vi "Periodic Tasks.vi"(8 "error in":errorcluster) -> ()   [LabVIEW 2016]
doc: "This VI runs in parallel to other tasks. It can contain as many user-defined periodic loops as you need. These can carry out PID or other sorts of timed response."
uses:
  <vilib>/Rock Robotics/WPI/Solenoid/WPI_SolenoidValue.ctl
  <vilib>/Rock Robotics/WPI/Utilities/WPI_GetSetVariantRefNum.vi
  Robot Global Data.vi
  <vilib>/addons/control/pid/pid.llb/PID (DBL).vi
  <vilib>/Rock Robotics/WPI/RobotDrive/WPI_RobotDriveMecanumDrive_Cartesian.vi
  <vilib>/Rock Robotics/WPI/Solenoid/WPI_SolenoidSetEnum.vi
  <vilib>/Rock Robotics/Network Tables/NT Read Number.vi
  <vilib>/Rock Robotics/Network Tables/NT Write Boolean.vi
  <vilib>/Rock Robotics/Network Tables/NT Write Number.vi
  <vilib>/Rock Robotics/Network Tables/NT Read Numeric Array.vi
  navX Library v2/navX Library v2.lvlib
  <vilib>/addons/control/pid/NI_PID_pid.lvlib
panel:
  out "timeSaved convey":i32
  out "timeSaved gears":i32
  out "encXsaved":dbl
  out "encYsaved":dbl
  out "voltage dash":dbl=12.55
  out "shooting far":bool
  out "shooting close":bool
  out "kill compress shoot":bool
  out "Pitch":dbl=0.2
  out "target angle":dbl=-4.022499999999997
  in  "cam FOV":dbl=34.0 format="%#_13g"
  out "YavSaved":dbl=-21.13
  in  "min thresh":dbl=5e-05 format="%#_13g"
  in  "add if slow":dbl=0.005 format="%#_13g"
  in  "add if fast":dbl format="%#_13g"
  out "turnSpeedSlow working":dbl=0.18
  out "aimState":i32
  out "leftOrRight":dbl=1.0
  out "aimBot":dbl
  in  "SEQ Retainer Open":bool
  in  "Gear Shover":bool
  in  "Ramp-Up":dbl format="%#_13g"
  out "Shooter Speed":dbl=-0.0
  out "trim close":dbl=0.9968503937007874
  out "trim far":dbl=1.0
  out "timeSaved 2":i32=29435
  out "timeSaved":i32=46200
  in  "Slews":cluster{"slewX":dbl, "slewY":dbl, "slewZ":dbl}={"slewX"=0.2, "slewY"=0.2, "slewZ"=0.15}
  # "ANYTHING AND EVERYTHING AUTOAIM"
  # "DRIVE STUFF"
  # "BALL STUFF"
  # "GEAR STUFF"
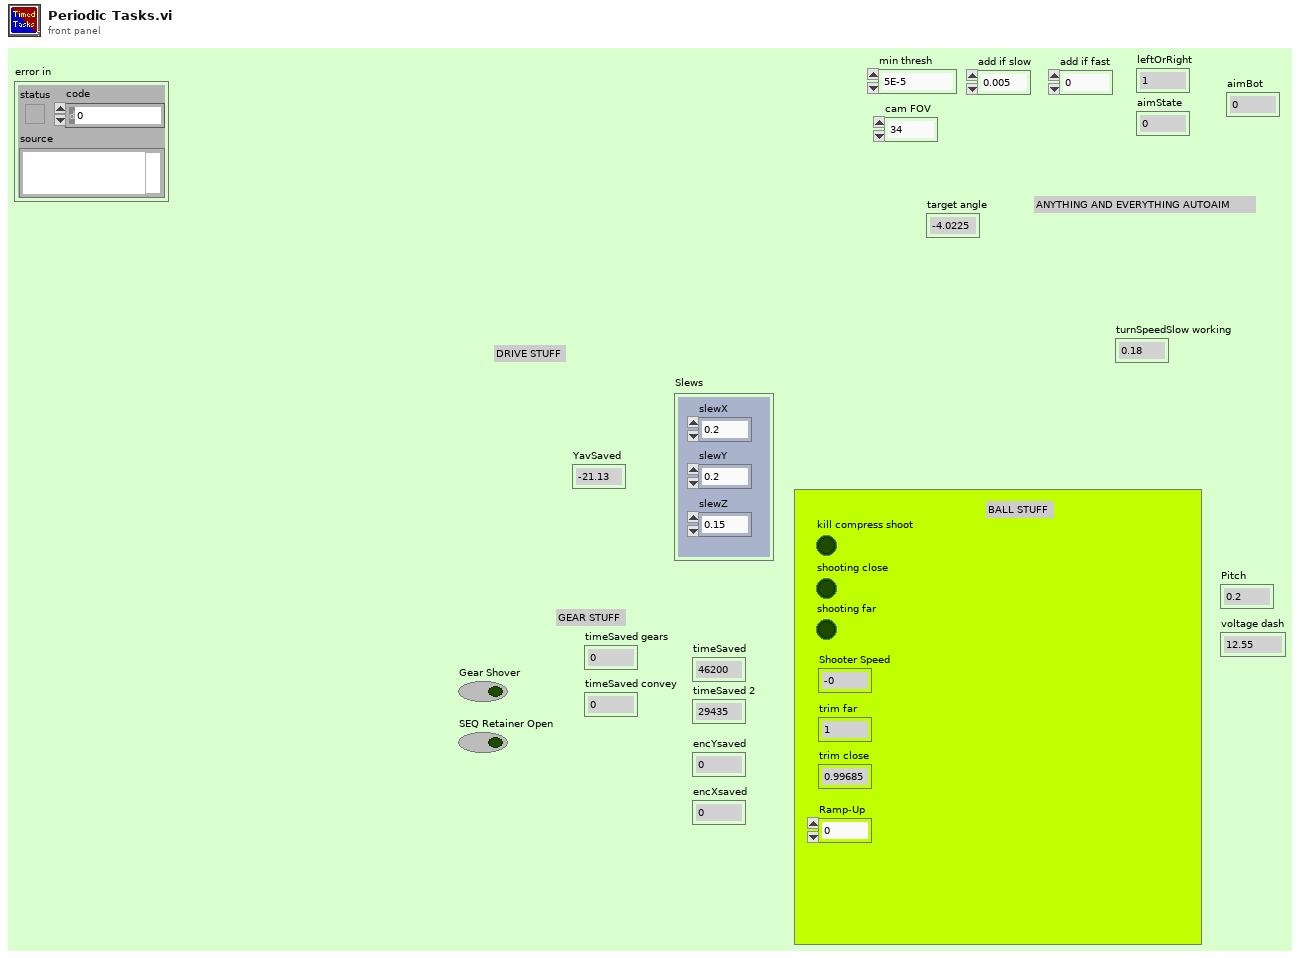
[diagram p1: front panel]
types:
  T1 = typedef "WPI_MotorControlDeviceRef.ctl" = cluster{"DeviceStatus":errorcluster, "Type":T2, "PWM":cluster{"PWM Channel":T3, "DeadBand":T4}, "CAN":cluster{"Device Number":u8, "SetOutput VI Ref":variant, "GetOutput VI Ref":variant, "Enable VI Ref":variant, "Disable VI Ref":variant, "Data":variant}, "Invert":bool}
  T2 = typedef "WPI_MotorControlType.ctl" = enum16{"PWM", "CAN"}
  T3 = typedef "FPGA_DIOPWMChannel.ctl" = enum8{"PWM 0", "PWM 1", "PWM 2", "PWM 3", "PWM 4", "PWM 5", "PWM 6", "PWM 7", "PWM 8", "PWM 9", "PWM MXP 0", "PWM MXP 1", "PWM MXP 2", "PWM MXP 3", "PWM MXP 4", "PWM MXP 5", "PWM MXP 6", "PWM MXP 7", "PWM MXP 8", "PWM MXP 9", "Invalid"}
  T4 = typedef "WPI_PWMDeadband.ctl" = cluster{"Name":string, "maxPositivePwm":i32, "minPositivePwm":i32, "centerPwm":i32, "maxNegativePwm":i32, "minNegativePwm":i32, "angularRange":u16}
  T5 = typedef "WPI_SolenoidDevRef.ctl" = cluster{"DevStatus":errorcluster, "Pneumatics Control Module":u8, "Forward Solenoid Channel":T6, "Reverse Solenoid Channel":T6}
  T6 = typedef "WPI_SolenoidChannel.ctl" = enum8{"Solenoid 0", "Solenoid 1", "Solenoid 2", "Solenoid 3", "Solenoid 4", "Solenoid 5", "Solenoid 6", "Solenoid 7", "Invalid"}
  T7 = typedef "WPI_CompressorDevRef.ctl" = cluster{"DevStatus":errorcluster, "Pneumatics Control Module":u8}
  T8 = typedef "WPI_ServoDeviceRef.ctl" = cluster{"DeviceStatus":errorcluster, "PWM Channel":T3, "DeadBand":T4}
  T9 = typedef "WPI_RobotDriveDevRef.ctl" = cluster{"DevStatus":errorcluster, "Motors[]":T1[], "Square Inputs":bool, "Max Output":dbl}
  T10 = typedef "navX Library v2.lvlib/Z900_navX_DeviceTypeDef.ctl" = cluster{"Interface":cluster{"Protocol":T11, "Update Rate (4Hz-100Hz)":u8, "navX Open TypeDef":variant}, "Notify Packet":refnum<notifier>, "Loop VI Refnum":refnum<vi>, "Ready to Close Occurrence Refnum":refnum<k4>}
  T11 = typedef "navX Library v2.lvlib/Z900_navX_ProtocolTypeDef.ctl" = enum16{"SERIAL", "I2C", "SPI"}
  T12 = typedef "WPI_SolenoidValue.ctl" = enum16{"Off", "On", "Forward", "Reverse"}
  T13 = typedef "WPI_EncoderDevRef.ctl" = cluster{"DevStatus":errorcluster, "EncoderIndex":T14, "CounterIndex":T15, "DistancePerCount":dbl, "Decoding Type":T16}
  T14 = typedef "FPGA_EncoderIdx.ctl" = enum8{"Enc 0", "Enc 1", "Enc 2", "Enc 3", "Enc 4", "Enc 5", "Enc 6", "Enc 7", "Invalid"}
  T15 = typedef "FPGA_CounterCtrSystemIndex.ctl" = enum8{"Ctr 0", "Ctr 1", "Ctr 2", "Ctr 3", "Ctr 4", "Ctr 5", "Ctr 6", "Ctr 7", "Invalid"}
  T16 = typedef "WPI_EncoderType.ctl" = enum16{"1x", "2x", "4x"}
  T17 = typedef "WPI_DriverStationRobotMode2.ctl" = enum16{"Autonomous Disabled", "Autonomous Enabled", "Teleop Disabled", "Teleop Enabled", "Disconnected", "Finish", "Test Disabled", "Test Enabled", "Emergency Stopped"}
  T18 = cluster{"proportional gain (Kc)":dbl, "integral time (Ti, min)":dbl, "derivative time (Td, min)":dbl}
  T19 = cluster{"Yaw":dbl, "Roll":dbl, "Pitch":dbl, "Heading":dbl, "Fused Heading":dbl}
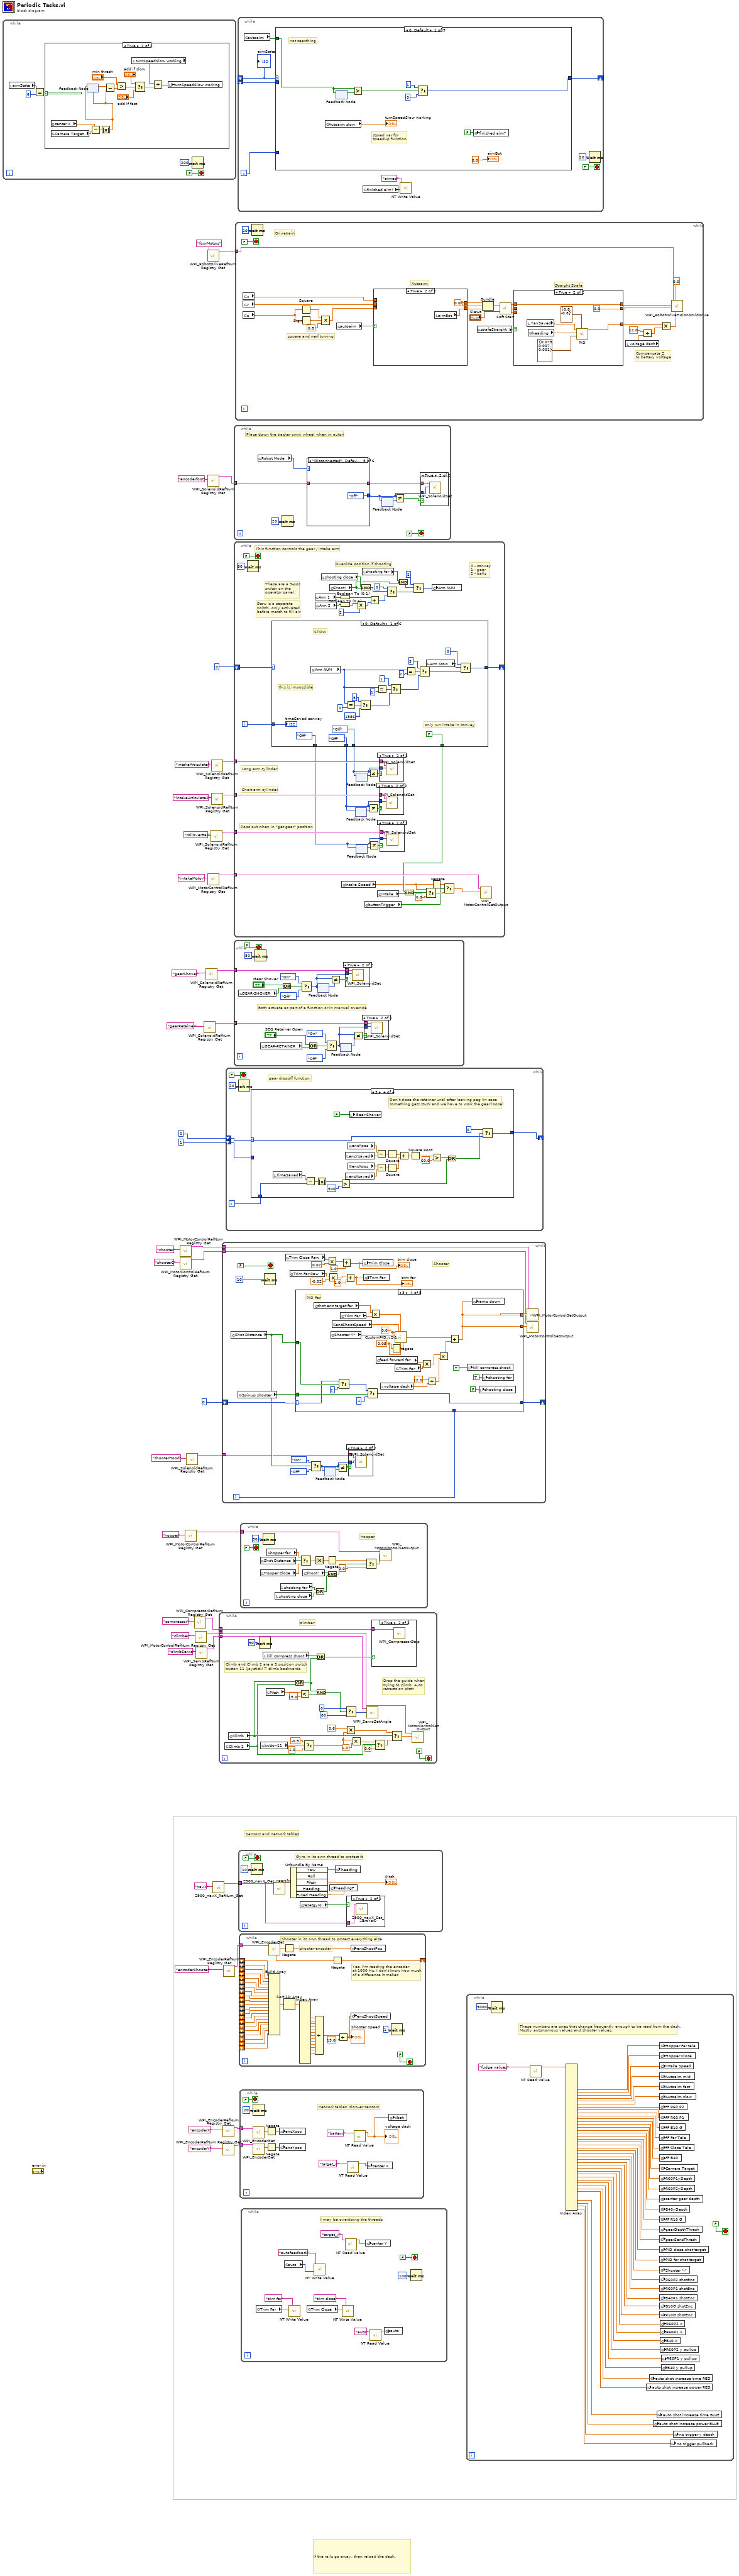
[diagram p0: block diagram]
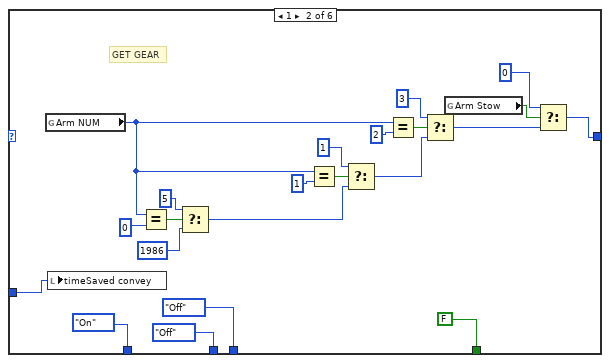
[diagram p5: hidden frame]
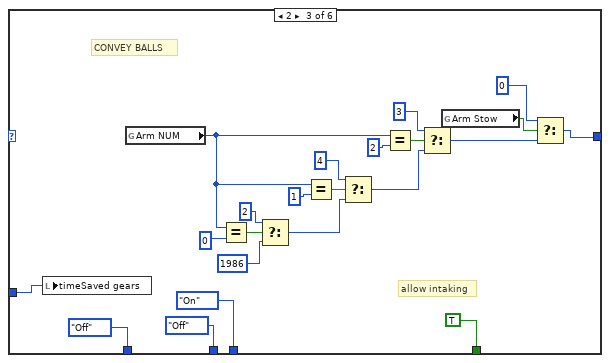
[diagram p6: hidden frame]
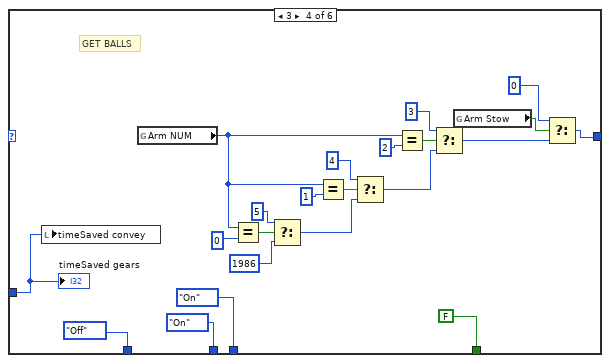
[diagram p7: hidden frame]
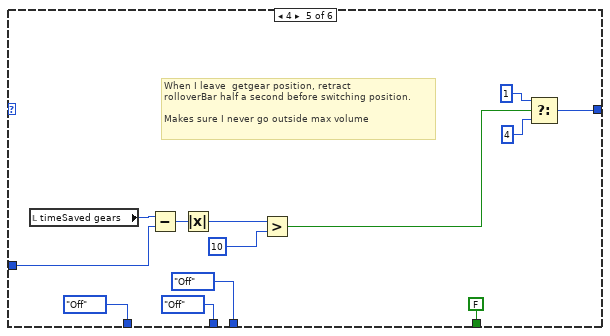
[diagram p8: hidden frame]
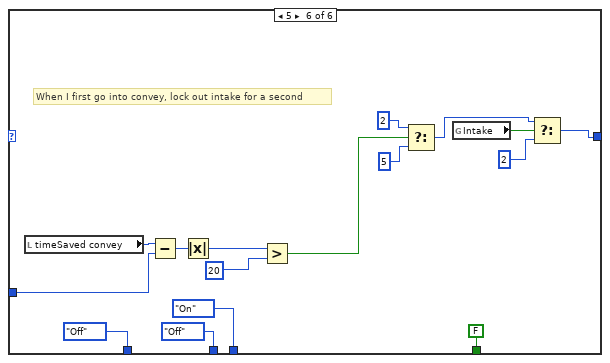
[diagram p9: hidden frame]
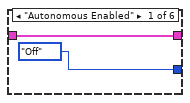
[diagram p11: hidden frame]
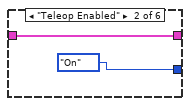
[diagram p12: hidden frame]
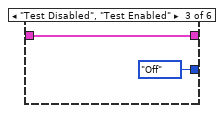
[diagram p13: hidden frame]
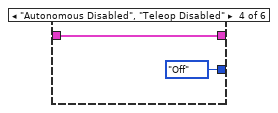
[diagram p14: hidden frame]
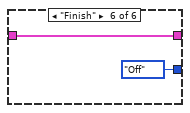
[diagram p15: hidden frame]
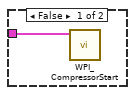
[diagram p17: hidden frame]
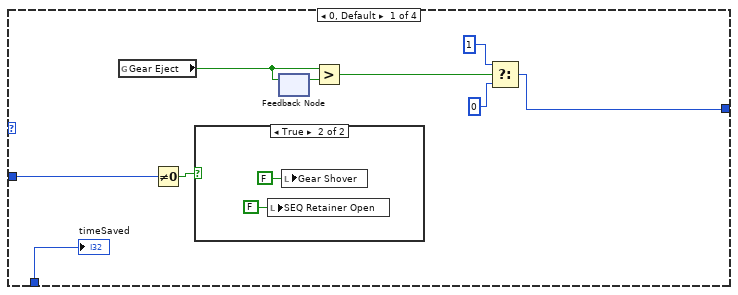
[diagram p18: hidden frame]
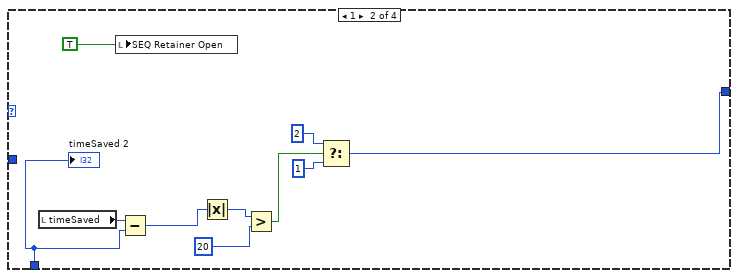
[diagram p20: hidden frame]
diagram:
  # "Sensors and network tables"
  # "If the rails go away, then reload the dash."
  n1 = while {
    stop <- FALSE stop-if-true
    n2 = local read "aimState"() -> (w45:i32)
    n3 = Equal?(x=w45, y=6) -> (x = y?=w43:bool)
    n4 = case shown="True" w43 {
      frame False {
      }
      frame True {
        n5 = global read "Robot Global Data.vi" "center X"() -> (w60:dbl)
        n6 = global read "Robot Global Data.vi" "Camera Target"() -> (w48:dbl)
        n7 = Subtract(x=w60, y=w48) -> (x-y=w50:dbl)
        n8 = Absolute Value(x=w50) -> (abs(x)=w49:dbl)
        n9 = feedback #1(w49) -> (w58:dbl)
        n10 = feedback-in #1(w49) -> ()
        n11 = Subtract(x=w58, y=w49) -> (x-y=w57:dbl)
        n12 = Greater?(x="min thresh", y=w57) -> (0:w55:bool)
        n13 = local read "turnSpeedSlow working"() -> (w52:dbl)
        n14 = Select(t="add if slow", s=w55, f="add if fast") -> (s? t:f=w53:dbl)
        n15 = Add(x=w52, y=w53) -> (x+y=w51:dbl)
        n16 = local write "turnSpeedSlow working"(w51) -> ()
      }
    }
    n17 = Wait (ms)(milliseconds to wait=u32 200) -> ()  [unwired: 1 out]
  }
  n18 = call <vilib>:"WPI_MotorControlRefNum Registry Get.vi"("refnum name"="shooter") -> ("MotorControlDevRef"=w31:T1)  [unwired: 9 in, 1 out]
  n19 = call <vilib>:"WPI_MotorControlRefNum Registry Get.vi"("refnum name"="shooter2") -> ("MotorControlDevRef"=w30:T1)  [unwired: 9 in, 1 out]
  n20 = call <vilib>:"WPI_MotorControlRefNum Registry Get.vi"("refnum name"="hopper") -> ("MotorControlDevRef"=w28:T1)  [unwired: 9 in, 1 out]
  n21 = call <vilib>:"WPI_SolenoidRefNum Registry Get.vi"("refnum name"="shooterHood") -> ("SolenoidDevRef"=w32:T5)  [unwired: 9 in, 1 out]
  n22 = call <vilib>:"WPI_CompressorRefNum Registry Get.vi"("refnum name"="compressor") -> ("CompressorDevRef"=w1:T7)  [unwired: 9 in, 1 out]
  n23 = call <vilib>:"WPI_MotorControlRefNum Registry Get.vi"("refnum name"="climber") -> ("MotorControlDevRef"=w24:T1)  [unwired: 9 in, 1 out]
  n24 = call <vilib>:"WPI_ServoRefNum Registry Get.vi"("refnum name"="climbServo") -> ("ServoDeviceRef"=w14:T8)  [unwired: 9 in, 1 out]
  n25 = call <vilib>:"WPI_SolenoidRefNum Registry Get.vi"("refnum name"="gearRetainer") -> ("SolenoidDevRef"=w37:T5)  [unwired: 9 in, 1 out]
  n26 = call <vilib>:"WPI_SolenoidRefNum Registry Get.vi"("refnum name"="gearShover") -> ("SolenoidDevRef"=w38:T5)  [unwired: 9 in, 1 out]
  n27 = call <vilib>:"WPI_RobotDriveRefNum Registry Get.vi"("refnum name"="fourMotors") -> ("RobotDriveDevRef"=w41:T9)  [unwired: 1 in, 9 out]
  n28 = call <vilib>:"WPI_SolenoidRefNum Registry Get.vi"("refnum name"="encoderfoot") -> ("SolenoidDevRef"=w11:T5)  [unwired: 9 in, 1 out]
  n29 = call <vilib>:"WPI_MotorControlRefNum Registry Get.vi"("refnum name"="intakeMotor") -> ("MotorControlDevRef"=w4:T1)  [unwired: 9 in, 1 out]
  n30 = call <vilib>:"WPI_SolenoidRefNum Registry Get.vi"("refnum name"="rolloverBar") -> ("SolenoidDevRef"=w2:T5)  [unwired: 9 in, 1 out]
  n31 = call <vilib>:"WPI_SolenoidRefNum Registry Get.vi"("refnum name"="intakeArticulate") -> ("SolenoidDevRef"=w8:T5)  [unwired: 9 in, 1 out]
  n32 = call <vilib>:"WPI_SolenoidRefNum Registry Get.vi"("refnum name"="intakeArticulate2") -> ("SolenoidDevRef"=w6:T5)  [unwired: 9 in, 1 out]
  n33 = call "Z900_navX_RefNum_Get.vi"("refnum name"="navX") -> ("navX Device"=w22:T10)  [unwired: 9 in, 1 out]
  n34 = while {
    tunnel: w24 -> [w67]
    tunnel: w14 -> [w83]
    tunnel: w1 -> [w75]
    stop <- FALSE stop-if-true
    # "Drop the guide when\ntrying to climb. Auto\nretracts on pitch"
    # "Climb and Climb 2 are a 3 position switch\nbutton 11 (joystick) = climb backwards"
    # "climber"
    n35 = global read "Robot Global Data.vi" "Climb 2"() -> (w64:bool)
    n36 = global read "Robot Global Data.vi" "Climb"() -> (w63:bool)
    n37 = Wait (ms)(milliseconds to wait=u32 50) -> ()  [unwired: 1 out]
    n38 = global read "Robot Global Data.vi" "button11"() -> (w69:bool)
    n39 = local read "kill compress shoot"() -> (w66:bool)
    n40 = local read "Pitch"() -> (w79:dbl)
    n41 = Or(x=w63, y=w64) -> (x .or. y?=w65:bool)
    n42 = Less?(x=w79, y=15.0) -> (x < y?=w80:bool)
    n43 = Select(t=-0.5, s=w69, f=1.0) -> (s? t:f=w61:dbl)
    n44 = Or(x=w66, y=w65) -> (x .or. y?=w76:bool)
    n45 = And(x=w65, y=w80) -> (x .and. y?=w77:bool)
    n46 = Select(t=0 ("servo down angle"), s=w77, f=80 ("servo up angle")) -> (s? t:f=w84:i32)
    n47 = Multiply(x=0.6 ("climb slow"), y=w61) -> (x*y=w68:dbl)
    n48 = Multiply(x=w61, y=1.0 ("t")) -> (x*y=w71:dbl)
    n49 = call <vilib>:"WPI_ServoSetAngle.vi"("Angle"=w84, "ServoDeviceRef"=w83) -> ()  [unwired: 8 in, 2 out]
    n50 = case shown="True" w76 {
      tunnel: w75 -> [w89 w90]
      frame False {
        n51 = call <vilib>:"WPI_CompressorStart.vi"("CompressorDevRef"=w89) -> ()  [unwired: 9 in, 2 out]
      }
      frame True {
        n52 = call <vilib>:"WPI_CompressorStop.vi"("CompressorDevRef"=w90) -> ()  [unwired: 9 in, 2 out]
      }
    }
    n53 = Select(t=w71, s=w64, f=0.0) -> (s? t:f=w85:dbl)
    n54 = Select(t=w68, s=w63, f=w85) -> (s? t:f=w74:dbl)
    n55 = call <vilib>:"WPI_MotorControlSetOutput.vi"("Output"=w74, "MotorControlDevRef"=w67) -> ()  [unwired: 7 in, 3 out]
  }
  n56 = while {
    shift-right: [w113] -> _
    shift-left: 0 ("y") -> [w115]
    tunnel: w32 -> [w96]
    tunnel: w31 -> [w95]
    tunnel: w30 -> [w94]
    i -> [w91]
    stop <- FALSE stop-if-true
    # "Shooter"
    n57 = global read "Robot Global Data.vi" "Shot Distance"() -> (w97:bool)
    n58 = global read "Robot Global Data.vi" "Spinup shooter"() -> (w114:bool)
    n59 = Wait (ms)(milliseconds to wait=u32 10) -> ()  [unwired: 1 out]
    n60 = global read "Robot Global Data.vi" "Trim Close Raw"() -> (w104:dbl)
    n61 = global read "Robot Global Data.vi" "Trim Far Raw"() -> (w106:dbl)
    n62 = case shown="3" w115 {
      selector: w115 -> [_ _ w167 w193 _]
      tunnel: w114 -> [w125 w143 w171 w192 _]
      tunnel: [w126 w139 w165 w191 w203] -> w113
      tunnel: [w122 w133 w156 w181 w200] -> w112
      tunnel: [w122 w133 w156 w181 w200] -> w111
      tunnel: w97 -> [_ w129 w168 w195 _]
      tunnel: w91 -> [_ _ _ _ _]
      frame 0, Default {
        w120 = FALSE ("shooting far")
        w122 = 0.0
        # "1"
        # "Reset Ramp to 0"
        # "Shooter-off"
        n63 = local write "Ramp-Up"(0.0 ("Power")) -> ()
        n64 = Select(t=1 ("f"), s=w125, f=0 ("y")) -> (s? t:f=w126:i32)
        "kill compress shoot" <- FALSE ("kill compress shoot")
        "shooting close" <- w120
        "shooting far" <- w120
      }
      frame 1 {
        # "Limit shooter spinup\n(should take ~1 sec"
        n65 = global read "Robot Global Data.vi" "FF Close Tele"() -> (w132:dbl)
        n66 = global read "Robot Global Data.vi" "feed forward far"() -> (w130:dbl)
        n67 = Add(x=0.01, y="Ramp-Up") -> (x+y=w133:dbl)
        n68 = local write "Ramp-Up"(w133) -> ()
        n69 = Select(t=w130, s=w129, f=w132) -> (s? t:f=w131:dbl)
        n70 = Select(t=1 ("f"), s=w143, f=4 ("y")) -> (s? t:f=w141:i32)
        n71 = Greater Or Equal?(x=w133, y=w131) -> (x >= y?=w140:bool)
        n72 = Select(t=3 ("y"), s=w129, f=2 ("y")) -> (s? t:f=w134:i32)
        n73 = Select(t=w134, s=w140, f=w141) -> (s? t:f=w139:i32)
        n74 = global write "Robot Global Data.vi" "ramp down"(w133) -> ()
        n75 = local write "kill compress shoot"(TRUE ("kill compress shoot")) -> ()
      }
      frame 2 {
        w147 = 0.0 ("Kp")
        w145 = 0.05 ("Max Ouput")
        # "PID Close"
        n76 = global read "Robot Global Data.vi" "PID close shot target"() -> (w152:dbl)
        n77 = global read "Robot Global Data.vi" "Shooter \"i\""() -> (w153:dbl)
        n78 = Select(t=3, s=w168, f=w167) -> (s? t:f=w166:i32)
        n79 = global read "Robot Global Data.vi" "Trim Close"() -> (w161:dbl)
        n80 = global read "Robot Global Data.vi" "encShootSpeed"() -> (w150:dbl)
        n81 = Select(t=w166, s=w171, f=4) -> (s? t:f=w165:i32)
        n82 = global read "Robot Global Data.vi" "FF Close Tele"() -> (w154:dbl)
        n83 = global read "Robot Global Data.vi" "Trim Close"() -> (w158:dbl)
        n84 = Multiply(x=w152, y=w161) -> (x*y=w160:dbl)
        n85 = local read "voltage dash"() -> (w155:dbl)
        n86 = Negate(x=w145) -> (-x=w146:dbl)
        n87 = call "CustomPID_v2.1.vi"("Kp"=w147, "Process Variable"=w150, "Goal"=w160, "Ki"=w153, "Kd"=w147, "Max Ouput"=w145, "Min Output"=w146) -> ("Command"=w159:dbl)  [unwired: 6 in, 2 out]
        n88 = Multiply(x=w154, y=w158) -> (x*y=w157:dbl)
        n89 = Divide(x=12.0, y=w155) -> (x/y=w163:dbl)
        n90 = Multiply(x=w157, y=w163) -> (x*y=w162:dbl)
        n91 = Add(x=w159, y=w162) -> (x+y=w156:dbl)
        n92 = local write "kill compress shoot"(TRUE ("kill compress shoot")) -> ()
        n93 = global write "Robot Global Data.vi" "ramp down"(w156) -> ()
        n94 = local write "shooting far"(FALSE ("shooting far")) -> ()
        n95 = local write "shooting close"(TRUE ("shooting close")) -> ()
      }
      frame 3 {
        w174 = 0.0 ("Kp")
        w172 = 0.05 ("Max Ouput")
        # "PID Far"
        n96 = global read "Robot Global Data.vi" "shot enc target far"() -> (w177:dbl)
        n97 = global read "Robot Global Data.vi" "Shooter \"i\""() -> (w179:dbl)
        n98 = global read "Robot Global Data.vi" "encShootSpeed"() -> (w185:dbl)
        n99 = Select(t=w193, s=w195, f=2 ("t")) -> (s? t:f=w196:i32)
        n100 = global read "Robot Global Data.vi" "Trim Far"() -> (w198:dbl)
        n101 = Select(t=w196, s=w192, f=4) -> (s? t:f=w191:i32)
        n102 = Multiply(x=w177, y=w198) -> (x*y=w186:dbl)
        n103 = global read "Robot Global Data.vi" "feed forward far"() -> (w182:dbl)
        n104 = local read "voltage dash"() -> (w180:dbl)
        n105 = Negate(x=w172) -> (-x=w173:dbl)
        n106 = call "CustomPID_v2.1.vi"("Kp"=w174, "Process Variable"=w185, "Goal"=w186, "Ki"=w179, "Kd"=w174, "Max Ouput"=w172, "Min Output"=w173) -> ("Command"=w187:dbl)  [unwired: 6 in, 2 out]
        n107 = global read "Robot Global Data.vi" "Trim Far"() -> (w184:dbl)
        n108 = Multiply(x=w182, y=w184) -> (x*y=w183:dbl)
        n109 = Divide(x=12.0, y=w180) -> (x/y=w189:dbl)
        n110 = Multiply(x=w183, y=w189) -> (x*y=w188:dbl)
        n111 = Add(x=w187, y=w188) -> (x+y=w181:dbl)
        n112 = local write "kill compress shoot"(TRUE ("kill compress shoot")) -> ()
        n113 = global write "Robot Global Data.vi" "ramp down"(w181) -> ()
        n114 = local write "shooting close"(FALSE ("shooting close")) -> ()
        n115 = local write "shooting far"(TRUE ("shooting far")) -> ()
      }
      frame 4 {
        # "With coast mode this is probably unecessary, but I left it in because I don't want to risk it\nI mean, we do cut the shooter abrubptly at the end of auto,="
        n116 = global read "Robot Global Data.vi" "ramp down"() -> (w201:dbl)
        n117 = Add(x=-0.002, y=w201) -> (x+y=w200:dbl)
        n118 = global write "Robot Global Data.vi" "ramp down"(w200) -> ()
        n119 = Less Or Equal To 0?(x=w200) -> (x <= 0?=w202:bool)
        n120 = Select(t=0 ("f"), s=w202, f=4 ("y")) -> (s? t:f=w203:i32)
        n121 = local write "kill compress shoot"(FALSE ("kill compress shoot")) -> ()
      }
    }
    n122 = Select(t=WPI_SolenoidValue."On" ("Value"), s=w97, f=WPI_SolenoidValue."Off" ("Value")) -> (s? t:f=w102:T12)
    n123 = feedback #2() -> (w100:T12)  [unwired: 1 in]
    n124 = feedback-in #2(w102) -> ()
    n125 = Multiply(x=w104, y=0.02 ("value")) -> (x*y=w107:dbl)
    n126 = Multiply(x=w106, y=-0.02 ("value")) -> (x*y=w110:dbl)
    n127 = Not Equal?(x=w102, y=w100) -> (x != y?=w101:bool)
    n128 = Add(x=w107, y=1.0) -> (x+y=w92:dbl)
    "trim close" <- w92
    n129 = Add(x=w110, y=1.0) -> (x+y=w93:dbl)
    "trim far" <- w93
    n130 = case shown="True" w101 {
      tunnel: w102 -> [_ w119]
      tunnel: w96 -> [_ w118]
      frame False {
      }
      frame True {
        n131 = call-poly <vilib>:"WPI_SolenoidSet.vi"("Value"=w119, "SolenoidDevRef"=w118) -> ()  [unwired: 8 in, 2 out]
      }
    }
    n132 = global write "Robot Global Data.vi" "Trim Close"(w92) -> ()
    n133 = global write "Robot Global Data.vi" "Trim Far"(w93) -> ()
    n134 = call <vilib>:"WPI_MotorControlSetOutput.vi"("Output"=w112, "MotorControlDevRef"=w95) -> ()  [unwired: 7 in, 3 out]
    n135 = call <vilib>:"WPI_MotorControlSetOutput.vi"("Output"=w111, "MotorControlDevRef"=w94) -> ()  [unwired: 7 in, 3 out]
  }
  n136 = call <vilib>:"WPI_EncoderRefNum Registry Get.vi"("refnum name"="encoderX") -> ("EncoderDevRef"=w18:T13)  [unwired: 9 in, 1 out]
  n137 = call <vilib>:"WPI_EncoderRefNum Registry Get.vi"("refnum name"="encoderY") -> ("EncoderDevRef"=w16:T13)  [unwired: 9 in, 1 out]
  n138 = call <vilib>:"WPI_EncoderRefNum Registry Get.vi"("refnum name"="encoderShooter") -> ("EncoderDevRef"=w20:T13)  [unwired: 9 in, 1 out]
  n139 = while {
    shift-right: [w209] -> _
    shift-left: 0 ("f") -> [w210]
    shift-left: 1 ("f") -> [w207]
    i -> [w208]
    stop <- FALSE stop-if-true
    # "gear dropoff function"
    n140 = Wait (ms)(milliseconds to wait=u32 20) -> ()  [unwired: 1 out]
    n141 = case shown="3" w210 {
      selector: w210 -> [_ _ w245 w263]
      tunnel: [w219 w225 w242 w262] -> w209
      tunnel: w208 -> [w216 w224 w236 w248]
      tunnel: w207 -> [w217 _ _ _]
      frame 0, Default {
        n142 = global read "Robot Global Data.vi" "Gear Eject"() -> (w213:bool)
        n143 = Not Equal To 0?(x=w217) -> (x != 0?=w218:bool)
        n144 = case shown="True" w218 {
          frame False {
          }
          frame True {
            n145 = local write "SEQ Retainer Open"(FALSE ("Gear Retainer")) -> ()
            n146 = local write "Gear Shover"(FALSE ("Gear Shover")) -> ()
          }
        }
        n147 = feedback #3() -> (w215:bool)  [unwired: 1 in]
        n148 = feedback-in #3(w213) -> ()
        n149 = Greater?(x=w213, y=w215) -> (0:w214:bool)
        n150 = Select(t=1, s=w214, f=0) -> (s? t:f=w219:i32)
        "timeSaved" <- w216
      }
      frame 1 {
        n151 = local read "timeSaved"() -> (w233:i32)
        n152 = local write "SEQ Retainer Open"(TRUE ("Gear Retainer")) -> ()
        n153 = Subtract(x=w233, y=w224) -> (x-y=w228:i32)
        n154 = Absolute Value(x=w228) -> (abs(x)=w227:i32)
        n155 = Greater?(x=w227, y=20 ("open retainer time")) -> (0:w230:bool)
        n156 = Select(t=2, s=w230, f=1) -> (s? t:f=w225:i32)
        "timeSaved 2" <- w224
      }
      frame 2 {
        n157 = local read "timeSaved 2"() -> (w241:i32)
        n158 = local write "Gear Shover"(TRUE ("Gear Shover")) -> ()
        n159 = local write "timeSaved"(w236) -> ()
        n160 = Subtract(x=w241, y=w236) -> (x-y=w238:i32)
        n161 = Absolute Value(x=w238) -> (abs(x)=w239:i32)
        n162 = Greater?(x=w239, y=20 ("drop gear time")) -> (0:w243:bool)
        n163 = Select(t=3, s=w243, f=w245) -> (s? t:f=w242:i32)
        n164 = global read "Robot Global Data.vi" "encYpos"() -> (→"encYsaved":dbl)
        n165 = global read "Robot Global Data.vi" "encXpos"() -> (→"encXsaved":dbl)
      }
      frame 3 {
        # "Don't close the retainer until after leaving peg (in case\nsomething gets stuck and we have to work the gear loose)"
        n166 = local read "timeSaved"() -> (w268:i32)
        n167 = Subtract(x=w268, y=w248) -> (x-y=w267:i32)
        n168 = Absolute Value(x=w267) -> (abs(x)=w266:i32)
        n169 = Greater?(x=w266, y=500) -> (0:w247:bool)
        n170 = local read "encYsaved"() -> (w259:dbl)
        n171 = local read "encXsaved"() -> (w257:dbl)
        n172 = global read "Robot Global Data.vi" "encYpos"() -> (w260:dbl)
        n173 = global read "Robot Global Data.vi" "encXpos"() -> (w258:dbl)
        n174 = local write "Gear Shover"(FALSE ("SEQ Retainer Open")) -> ()
        n175 = Subtract(x=w260, y=w259) -> (x-y=w256:dbl)
        n176 = Subtract(x=w258, y=w257) -> (x-y=w255:dbl)
        n177 = Square(x=w256) -> (x^2=w254:dbl)
        n178 = Square(x=w255) -> (x^2=w253:dbl)
        n179 = Add(x=w254, y=w253) -> (x+y=w252:dbl)
        n180 = Square Root(x=w252) -> (sqrt(x)=w251:dbl)
        n181 = Greater?(x=w251, y=60.0) -> (0:w249:bool)
        n182 = Or(x=w249, y=w247) -> (x .or. y?=w246:bool)
        n183 = Select(t=0, s=w246, f=w263) -> (s? t:f=w262:i32)
      }
    }
  }
  n184 = while {
    tunnel: w11 -> [w276]
    stop <- FALSE stop-if-true
    # "Place down the tracker omni wheel when in auton"
    n185 = global read "Robot Global Data.vi" "Robot Mode"() -> (w273:T17)
    n186 = Wait (ms)(milliseconds to wait=u32 20) -> ()  [unwired: 1 out]
    n187 = case shown="\"Disconnected\", Default" w273 {
      tunnel: w276 -> [w280 w282 w284 w286 w288 w290]
      tunnel: [w280 w282 w284 w286 w288 w290] -> w272
      tunnel: [WPI_SolenoidValue."Off" ("Value") WPI_SolenoidValue."On" ("Value") WPI_SolenoidValue."Off" ("Value") WPI_SolenoidValue."Off" ("Value") WPI_SolenoidValue."Off" ("Value") WPI_SolenoidValue."Off" ("Value")] -> w270
      frame "Autonomous Enabled" {
      }
      frame "Teleop Enabled" {
      }
      frame "Test Disabled", "Test Enabled" {
      }
      frame "Autonomous Disabled", "Teleop Disabled" {
      }
      frame "Disconnected", Default {
      }
      frame "Finish" {
      }
    }
    n188 = feedback #4() -> (w271:T12)  [unwired: 1 in]
    n189 = feedback-in #4(w270) -> ()
    n190 = Not Equal?(x=w270, y=w271) -> (x != y?=w269:bool)
    n191 = case shown="True" w269 {
      tunnel: w272 -> [_ w278]
      tunnel: w270 -> [_ w277]
      frame False {
      }
      frame True {
        n192 = call-poly <vilib>:"WPI_SolenoidSet.vi"("Value"=w277, "SolenoidDevRef"=w278) -> ()  [unwired: 8 in, 2 out]
      }
    }
  }
  n193 = while {
    shift-right: [w312] -> _
    shift-left: 0 -> [w333]
    tunnel: w8 -> [w327]
    tunnel: w6 -> [w326]
    tunnel: w4 -> [w308]
    tunnel: w2 -> [w303]
    i -> [w306]
    stop <- FALSE stop-if-true
    # "Stow is a seperate\nswitch, only activated\nbefore match to fill air"
    # "Pops out when in \"get gear\" position"
    # "This function controls the gear / intake arm"
    # "0 - convey\n1 - gear\n2 - balls"
    # "Override position if shooting"
    # "These are a 3-pos\nswitch on the\noperator panel."
    # "Short arm cylinder"
    # "Long arm cylinder"
    n194 = Wait (ms)(milliseconds to wait=u32 50) -> ()  [unwired: 1 out]
    n195 = case shown="0, Default" w333 {
      tunnel: [WPI_SolenoidValue."Off" ("Value") WPI_SolenoidValue."Off" ("Value") WPI_SolenoidValue."On" ("Value") WPI_SolenoidValue."On" ("Value") WPI_SolenoidValue."Off" ("Value") WPI_SolenoidValue."On" ("Value")] -> w325
      tunnel: [WPI_SolenoidValue."Off" ("Value") WPI_SolenoidValue."Off" ("Value") WPI_SolenoidValue."Off" ("Value") WPI_SolenoidValue."On" ("Value") WPI_SolenoidValue."Off" ("Value") WPI_SolenoidValue."Off" ("Value")] -> w324
      tunnel: [w343 w363 w387 w409 w430 w444] -> w312
      tunnel: [FALSE FALSE TRUE FALSE FALSE FALSE] -> w296
      tunnel: w306 -> [w340 w362 w384 w406 w436 w452]
      tunnel: [WPI_SolenoidValue."Off" ("Value") WPI_SolenoidValue."On" ("Value") WPI_SolenoidValue."Off" ("Value") WPI_SolenoidValue."Off" ("Value") WPI_SolenoidValue."Off" ("Value") WPI_SolenoidValue."Off" ("Value")] -> w302
      frame 0, Default {
        # "only run intake in convey"
        # "this is impossible"
        # "STOW"
        n196 = global read "Robot Global Data.vi" "Arm NUM"() -> (w347:i16)
        n197 = Equal?(x=w347, y=i16 0) -> (x = y?=w358:bool)
        n198 = Select(t=5, s=w358, f=1986) -> (s? t:f=w352:i32)
        n199 = Equal?(x=w347, y=i16 1) -> (x = y?=w354:bool)
        n200 = Select(t=1, s=w354, f=w352) -> (s? t:f=w348:i32)
        n201 = Equal?(x=w347, y=i16 2) -> (x = y?=w350:bool)
        n202 = Select(t=3, s=w350, f=w348) -> (s? t:f=w344:i32)
        n203 = global read "Robot Global Data.vi" "Arm Stow"() -> (w345:bool)
        n204 = Select(t=0, s=w345, f=w344) -> (s? t:f=w343:i32)
        "timeSaved convey" <- w340
      }
      frame 1 {
        # "GET GEAR"
        n205 = global read "Robot Global Data.vi" "Arm NUM"() -> (w367:i16)
        n206 = local write "timeSaved convey"(w362) -> ()
        n207 = Equal?(x=w367, y=i16 0) -> (x = y?=w378:bool)
        n208 = Select(t=5, s=w378, f=1986) -> (s? t:f=w372:i32)
        n209 = Equal?(x=w367, y=i16 1) -> (x = y?=w374:bool)
        n210 = Select(t=1, s=w374, f=w372) -> (s? t:f=w368:i32)
        n211 = Equal?(x=w367, y=i16 2) -> (x = y?=w370:bool)
        n212 = Select(t=3, s=w370, f=w368) -> (s? t:f=w364:i32)
        n213 = global read "Robot Global Data.vi" "Arm Stow"() -> (w365:bool)
        n214 = Select(t=0, s=w365, f=w364) -> (s? t:f=w363:i32)
      }
      frame 2 {
        # "allow intaking"
        # "CONVEY BALLS"
        n215 = local write "timeSaved gears"(w384) -> ()
        n216 = global read "Robot Global Data.vi" "Arm NUM"() -> (w391:i16)
        n217 = Equal?(x=w391, y=i16 0) -> (x = y?=w402:bool)
        n218 = Select(t=2, s=w402, f=1986) -> (s? t:f=w396:i32)
        n219 = Equal?(x=w391, y=i16 1) -> (x = y?=w398:bool)
        n220 = Select(t=4, s=w398, f=w396) -> (s? t:f=w392:i32)
        n221 = Equal?(x=w391, y=i16 2) -> (x = y?=w394:bool)
        n222 = Select(t=3, s=w394, f=w392) -> (s? t:f=w388:i32)
        n223 = global read "Robot Global Data.vi" "Arm Stow"() -> (w389:bool)
        n224 = Select(t=0, s=w389, f=w388) -> (s? t:f=w387:i32)
      }
      frame 3 {
        # "GET BALLS"
        n225 = local write "timeSaved convey"(w406) -> ()
        n226 = global read "Robot Global Data.vi" "Arm NUM"() -> (w413:i16)
        n227 = Equal?(x=w413, y=i16 0) -> (x = y?=w424:bool)
        n228 = Select(t=5, s=w424, f=1986) -> (s? t:f=w418:i32)
        n229 = Equal?(x=w413, y=i16 1) -> (x = y?=w420:bool)
        n230 = Select(t=4, s=w420, f=w418) -> (s? t:f=w414:i32)
        n231 = Equal?(x=w413, y=i16 2) -> (x = y?=w416:bool)
        n232 = Select(t=3, s=w416, f=w414) -> (s? t:f=w410:i32)
        n233 = global read "Robot Global Data.vi" "Arm Stow"() -> (w411:bool)
        n234 = Select(t=0, s=w411, f=w410) -> (s? t:f=w409:i32)
        "timeSaved gears" <- w406
      }
      frame 4 {
        # "When I leave  getgear position, retract\nrolloverBar half a second before switching position.\n\nMakes sure I never go outside max volume"
        n235 = local read "timeSaved gears"() -> (w437:i32)
        n236 = Subtract(x=w437, y=w436) -> (x-y=w435:i32)
        n237 = Absolute Value(x=w435) -> (abs(x)=w434:i32)
        n238 = Greater?(x=w434, y=10 ("post gear delay")) -> (0:w432:bool)
        n239 = Select(t=1, s=w432, f=4) -> (s? t:f=w430:i32)
      }
      frame 5 {
        # "When I first go into convey, lock out intake for a second"
        n240 = local read "timeSaved convey"() -> (w453:i32)
        n241 = Subtract(x=w453, y=w452) -> (x-y=w451:i32)
        n242 = Absolute Value(x=w451) -> (abs(x)=w450:i32)
        n243 = Greater?(x=w450, y=20 ("post convey delay")) -> (0:w448:bool)
        n244 = Select(t=2, s=w448, f=5) -> (s? t:f=w442:i32)
        n245 = global read "Robot Global Data.vi" "Intake"() -> (w443:bool)
        n246 = Select(t=w442, s=w443, f=2) -> (s? t:f=w444:i32)
      }
    }
    n247 = global read "Robot Global Data.vi" "Arm 1"() -> (w315:bool)
    n248 = global read "Robot Global Data.vi" "Arm 2"() -> (w314:bool)
    n249 = local read "shooting close"() -> (w300:bool)
    n250 = global read "Robot Global Data.vi" "Shoot!"() -> (w297:bool)
    n251 = Boolean To (0,1)(Boolean=w315) -> (0, 1=w313:i16)
    n252 = Boolean To (0,1)(Boolean=w314) -> (0, 1=w317:i16)
    n253 = global read "Robot Global Data.vi" "Intake Speed"() -> (w291:dbl)
    n254 = feedback #5() -> (w329:T12)  [unwired: 1 in]
    n255 = feedback-in #5(w324) -> ()
    n256 = Multiply(x=w317, y=i16 2) -> (x*y=w316:i16)
    n257 = feedback #6() -> (w331:T12)  [unwired: 1 in]
    n258 = feedback-in #6(w325) -> ()
    n259 = feedback #7() -> (w305:T12)  [unwired: 1 in]
    n260 = feedback-in #7(w302) -> ()
    n261 = And(x=w300, y=w297) -> (x .and. y?=w301:bool)
    n262 = local read "shooting far"() -> (w299:bool)
    n263 = global read "Robot Global Data.vi" "buttonTrigger"() -> (w293:bool)
    n264 = Not Equal?(x=w324, y=w329) -> (x != y?=w328:bool)
    n265 = Not Equal?(x=w325, y=w331) -> (x != y?=w330:bool)
    n266 = Not Equal?(x=w302, y=w305) -> (x != y?=w304:bool)
    n267 = Add(x=w313, y=w316) -> (x+y=w323:i16)
    n268 = global read "Robot Global Data.vi" "Intake"() -> (w307:bool)
    n269 = case shown="True" w328 {
      tunnel: w324 -> [_ w337]
      tunnel: w326 -> [_ w336]
      frame False {
      }
      frame True {
        n270 = call-poly <vilib>:"WPI_SolenoidSet.vi"("Value"=w337, "SolenoidDevRef"=w336) -> ()  [unwired: 8 in, 2 out]
      }
    }
    n271 = case shown="True" w330 {
      tunnel: w325 -> [_ w338]
      tunnel: w327 -> [_ w339]
      frame False {
      }
      frame True {
        n272 = call-poly <vilib>:"WPI_SolenoidSet.vi"("Value"=w338, "SolenoidDevRef"=w339) -> ()  [unwired: 8 in, 2 out]
      }
    }
    n273 = case shown="True" w304 {
      tunnel: w302 -> [_ w335]
      tunnel: w303 -> [_ w334]
      frame False {
      }
      frame True {
        n274 = call-poly <vilib>:"WPI_SolenoidSet.vi"("Value"=w335, "SolenoidDevRef"=w334) -> ()  [unwired: 8 in, 2 out]
      }
    }
    n275 = Select(t=i16 0, s=w301, f=w323) -> (s? t:f=w320:i16)
    n276 = And(x=w299, y=w297) -> (x .and. y?=w298:bool)
    n277 = And(x=w296, y=w307) -> (x .and. y?=w310:bool)
    n278 = Select(t=i16 2, s=w298, f=w320) -> (s? t:f=w321:i16)
    n279 = Select(t=w291, s=w310, f=0.0) -> (s? t:f=w295:dbl)
    n280 = Negate(x=w291) -> (-x=w292:dbl)
    n281 = global write "Robot Global Data.vi" "Arm NUM"(w321) -> ()
    n282 = Select(t=w292, s=w293, f=w295) -> (s? t:f=w294:dbl)
    n283 = call <vilib>:"WPI_MotorControlSetOutput.vi"("Output"=w294, "MotorControlDevRef"=w308) -> ()  [unwired: 7 in, 3 out]
  }
  n284 = while {
    tunnel: w38 -> [w462]
    tunnel: w37 -> [w460]
    stop <- FALSE stop-if-true
    # "Both actuate as part of a function or in manual override"
    n285 = global read "Robot Global Data.vi" "GEAR-SHOVER"() -> (w466:bool)
    n286 = Wait (ms)(milliseconds to wait=u32 50) -> ()  [unwired: 1 out]
    n287 = global read "Robot Global Data.vi" "GEAR-RETAINER"() -> (w467:bool)
    n288 = Or(x="Gear Shover", y=w466) -> (x .or. y?=w470:bool)
    n289 = Select(t=WPI_SolenoidValue."On" ("Value"), s=w470, f=WPI_SolenoidValue."Off" ("Value")) -> (s? t:f=w461:T12)
    n290 = Or(x="SEQ Retainer Open", y=w467) -> (x .or. y?=w469:bool)
    n291 = feedback #8() -> (w464:T12)  [unwired: 1 in]
    n292 = feedback-in #8(w461) -> ()
    n293 = Select(t=WPI_SolenoidValue."On" ("Value"), s=w469, f=WPI_SolenoidValue."Off" ("Value")) -> (s? t:f=w457:T12)
    n294 = Not Equal?(x=w461, y=w464) -> (x != y?=w463:bool)
    n295 = feedback #9() -> (w459:T12)  [unwired: 1 in]
    n296 = feedback-in #9(w457) -> ()
    n297 = case shown="True" w463 {
      tunnel: w461 -> [_ w480]
      tunnel: w462 -> [_ w479]
      frame False {
      }
      frame True {
        n298 = call-poly <vilib>:"WPI_SolenoidSet.vi"("Value"=w480, "SolenoidDevRef"=w479) -> ()  [unwired: 8 in, 2 out]
      }
    }
    n299 = Not Equal?(x=w457, y=w459) -> (x != y?=w458:bool)
    n300 = case shown="True" w458 {
      tunnel: w460 -> [_ w478]
      tunnel: w457 -> [_ w477]
      frame False {
      }
      frame True {
        n301 = call-poly <vilib>:"WPI_SolenoidSet.vi"("Value"=w477, "SolenoidDevRef"=w478) -> ()  [unwired: 8 in, 2 out]
      }
    }
  }
  n302 = while {
    tunnel: w41 -> [w504]
    stop <- FALSE stop-if-true
    # "Compensate Z\nto battery voltage"
    # "Straight Strafe"
    # "Autoaim"
    # "Drivetrain"
    # "square and nerf turning"
    n303 = global read "Robot Global Data.vi" "x"() -> (w481:dbl)
    n304 = global read "Robot Global Data.vi" "y"() -> (w483:dbl)
    n305 = global read "Robot Global Data.vi" "z"() -> (w506:dbl)
    n306 = Wait (ms)(milliseconds to wait=u32 20) -> ()  [unwired: 1 out]
    n307 = Square(x=w506) -> (x^2=w502:dbl)
    n308 = Sign(1:w506) -> (0:w501:dbl)
    n309 = Compound Arithmetic op=MULTIPLY(w502, w501, 0.8 ("value")) -> (w482:dbl)
    n310 = global read "Robot Global Data.vi" "autoaim"() -> (w484:bool)
    n311 = case shown="True" w484 {
      tunnel: [w509 w512] -> w487
      tunnel: [w510 w513] -> w486
      tunnel: [w511 w513] -> w485
      tunnel: w481 -> [w511 _]
      tunnel: w483 -> [w510 _]
      tunnel: w482 -> [w509 _]
      frame False {
      }
      frame True {
        w513 = 0.0 ("x")
        n312 = local read "aimBot"() -> (w512:dbl)
      }
    }
    n313 = global read "Robot Global Data.vi" "strafeStraight"() -> (w495:bool)
    n314 = Bundle("x"=w485, "x"=w486, "aimBot"=w487) -> (w499:cluster{"x":dbl, "x":dbl, "aimBot":dbl})  [unwired: 1 in]
    n315 = call "Soft Start.vi"("Joysticks"=w499, "Slew Rates"="Slews") -> ("X-axis drive"=w498:dbl, "Y-axis drive"=w497:dbl, "Z-axis drive"=w496:dbl)
    n316 = case shown="True" w495 {
      tunnel: [w517 w518] -> w490
      tunnel: w498 -> [w517 w518]
      tunnel: [w516 0.0 ("Y-axis drive")] -> w489
      tunnel: w497 -> [w516 _]
      tunnel: [w515 w519] -> w488
      tunnel: w496 -> [w515 _]
      frame False {
        n317 = global read "Robot Global Data.vi" "heading"() -> (→"YavSaved":dbl)
      }
      frame True {
        n318 = local read "YavSaved"() -> (w521:dbl)
        n319 = global read "Robot Global Data.vi" "heading"() -> (w520:dbl)
        n320 = call-poly <vilib>:"PID.vi"("output range"=cluster{"output high":dbl, "output low":dbl} {"output high"=0.8, "output low"=-0.8}, "PID gains"=T18 {"proportional gain (Kc)"=0.075, "integral time (Ti, min)"=0.007, "derivative time (Td, min)"=0.001} ("PID Strafe Straight"), "process variable"=w520, "setpoint"=w521) -> ("output"=w519:dbl)  [unwired: 6 in, 1 out]
      }
    }
    n321 = local read "voltage dash"() -> (w491:dbl)
    n322 = Divide(x=12.0, y=w491) -> (x/y=w492:dbl)
    n323 = Multiply(x=w488, y=w492) -> (x*y=w493:dbl)
    n324 = call-poly <vilib>:"WPI_RobotDriveHolonomicDrive.vi"("Rotation"=w493, "Gyro Angle"=0.0, "Y"=w489, "X"=w490, "RobotDriveDevRef"=w504) -> ()  [unwired: 4 in, 3 out]
  }
  n325 = while {
    shift-right: [w532] -> _
    shift-left: _ -> [w530]
    shift-left: _ -> [w527]
    i -> [w528]
    stop <- FALSE stop-if-true
    n326 = global read "Robot Global Data.vi" "autoaim"() -> (w531:bool)
    n327 = case shown="0, Default" w530 {
      tunnel: w531 -> [w536 w553 w568 w589 w614]
      tunnel: [w540 w563 w581 w603 w610] -> w532
      tunnel: w528 -> [_ _ _ _ _]
      tunnel: w527 -> [_ _ w574 w598 w613]
      frame 0, Default {
        # "stored var for\nspeedup function"
        # "not searching"
        n328 = global read "Robot Global Data.vi" "Autoaim slow"() -> (→"turnSpeedSlow working":dbl)
        n329 = feedback #10() -> (w542:bool)  [unwired: 1 in]
        n330 = feedback-in #10(w536) -> ()
        n331 = Greater?(x=w536, y=w542) -> (0:w539:bool)
        n332 = Select(t=1, s=w539, f=0) -> (s? t:f=w540:i32)
        n333 = global write "Robot Global Data.vi" "finished aim?"(FALSE ("4?")) -> ()
        "aimBot" <- 0.0 ("aimBot")
      }
      frame 1 {
        # "7"
        # "If button released then\nbail-out to case 0."
        n334 = global read "Robot Global Data.vi" "Camera Target"() -> (w545:dbl)
        n335 = global read "Robot Global Data.vi" "center Y"() -> (w561:dbl)
        n336 = global read "Robot Global Data.vi" "center X"() -> (w551:dbl)
        n337 = global read "Robot Global Data.vi" "Camera Target"() -> (w544:dbl)
        n338 = Equal To 0?(x=w561) -> (x = 0?=w559:bool)
        n339 = Equal To 0?(x=w551) -> (x = 0?=w560:bool)
        n340 = Subtract(x=w551, y=w545) -> (x-y=w550:dbl)
        n341 = global read "Robot Global Data.vi" "center X"() -> (w556:dbl)
        n342 = Not And(1:w560, 2:w559) -> (0:w558:bool)
        n343 = Multiply(x=w550, y="cam FOV") -> (x*y=w547:dbl)
        n344 = global read "Robot Global Data.vi" "heading"() -> (w546:dbl)
        n345 = Subtract(x=w556, y=w544) -> (x-y=w555:dbl)
        n346 = Add(x=w547, y=w546) -> (x+y=→"target angle":dbl)
        n347 = Sign(1:w555) -> (0:→"leftOrRight":dbl)
        n348 = Not(x=w553) -> (.not. x?=w552:bool)
        n349 = Select(t=2, s=w558, f=1) -> (s? t:f=w557:i32)
        n350 = Select(t=0, s=w552, f=w557) -> (s? t:f=w563:i32)
      }
      frame 2 {
        # "camera - target"
        # "Build in 2.25 degrees for tire bounce back"
        # "Dont energize motors in first loop"
        # "If button released then\nbail-out to case 0."
        n351 = global read "Robot Global Data.vi" "heading"() -> (w567:dbl)
        n352 = local read "target angle"() -> (w566:dbl)
        n353 = Equal?(x=w574, y=1) -> (x = y?=w572:bool)
        n354 = Subtract(x=w566, y=w567) -> (x-y=w577:dbl)
        n355 = Sign(1:w577) -> (0:w578:dbl)
        n356 = Absolute Value(x=w577) -> (abs(x)=w579:dbl)
        n357 = Not(x=w568) -> (.not. x?=w569:bool)
        n358 = global read "Robot Global Data.vi" "Autoaim fast"() -> (w565:dbl)
        n359 = Less Or Equal?(x=w579, y=90.0 ("aim thresh fast to mid")) -> (x <= y?=w580:bool)
        n360 = local read "aimBot"() -> (w571:dbl)
        n361 = Multiply(x=w578, y=w565) -> (x*y=w576:dbl)
        n362 = Select(t=w571, s=w572, f=w576) -> (s? t:f=w575:dbl)
        n363 = local write "aimBot"(w575) -> ()
        n364 = Select(t=3, s=w580, f=2) -> (s? t:f=w583:i32)
        n365 = Select(t=0, s=w569, f=w583) -> (s? t:f=w581:i32)
      }
      frame 3 {
        # "Dont energize motors in first loop"
        # "If button released then\nbail-out to case 0."
        n366 = global read "Robot Global Data.vi" "heading"() -> (w588:dbl)
        n367 = local read "target angle"() -> (w587:dbl)
        n368 = Equal?(x=w598, y=2) -> (x = y?=w596:bool)
        n369 = Subtract(x=w587, y=w588) -> (x-y=w601:dbl)
        n370 = Not(x=w589) -> (.not. x?=w590:bool)
        n371 = global read "Robot Global Data.vi" "Autoaim mid"() -> (w586:dbl)
        n372 = Absolute Value(x=w601) -> (abs(x)=w602:dbl)
        n373 = Less Or Equal?(x=w602, y=30.0 ("aim thresh mid to slow")) -> (x <= y?=w592:bool)
        n374 = local read "aimBot"() -> (w595:dbl)
        n375 = Sign(1:w601) -> (0:w594:dbl)
        n376 = Multiply(x=w594, y=w586) -> (x*y=w600:dbl)
        n377 = Select(t=w595, s=w596, f=w600) -> (s? t:f=w599:dbl)
        n378 = local write "aimBot"(w599) -> ()
        n379 = Select(t=4, s=w592, f=3) -> (s? t:f=w605:i32)
        n380 = Select(t=0, s=w590, f=w605) -> (s? t:f=w603:i32)
      }
      frame 4 {
        # "Dont energize motors in first loop"
        # "If button released then\nbail-out to case 0."
        n381 = global read "Robot Global Data.vi" "heading"() -> (w612:dbl)
        n382 = local read "target angle"() -> (w611:dbl)
        n383 = Equal?(x=w613, y=3) -> (x = y?=w620:bool)
        n384 = Subtract(x=w611, y=w612) -> (x-y=w623:dbl)
        n385 = Absolute Value(x=w623) -> (abs(x)=w615:dbl)
        n386 = local read "turnSpeedSlow working"() -> (w616:dbl)
        n387 = Not(x=w614) -> (.not. x?=w608:bool)
        n388 = local read "aimBot"() -> (w619:dbl)
        n389 = Sign(1:w623) -> (0:w624:dbl)
        n390 = Multiply(x=w624, y=w616) -> (x*y=w622:dbl)
        n391 = Less Or Equal?(x=w615, y=0.5 ("aimTolerance 2")) -> (x <= y?=w607:bool)
        n392 = Select(t=w619, s=w620, f=w622) -> (s? t:f=w617:dbl)
        n393 = Or(x=w608, y=w607) -> (x .or. y?=w609:bool)
        n394 = Select(t=0, s=w609, f=6) -> (s? t:f=w610:i32)
        n395 = local write "aimBot"(w617) -> ()
      }
    }
    n396 = global read "Robot Global Data.vi" "finished aim?"() -> (w526:bool)
    n397 = call-poly <vilib>:"NT Write Value.vi"("Boolean"=w526, "Name"="aimed") -> ()  [unwired: 9 in, 1 out]
    n398 = Wait (ms)(milliseconds to wait=u32 20) -> ()  [unwired: 1 out]
    "aimState" <- w530
  }
  n399 = while {
    tunnel: w22 -> [w628]
    stop <- FALSE stop-if-true
    # "Gyro in its own thread to protect it"
    n400 = Wait (ms)(milliseconds to wait=u32 10) -> ()  [unwired: 1 out]
    n401 = call "Z900_navX_Get_YPRHfH.vi"("navX Device"=w628) -> ("YRPHfH"=w634:T19)  [unwired: 7 in, 3 out]
    n402 = Unbundle By Name(w634) -> ("Yaw"=w633:dbl, "Pitch"=→"Pitch":dbl, "Fused Heading"=w630:dbl)  [unwired: 2 out]
    n403 = global read "Robot Global Data.vi" "resetgyro"() -> (w629:bool)
    n404 = global write "Robot Global Data.vi" "headingF"(w630) -> ()
    n405 = global write "Robot Global Data.vi" "heading"(w633) -> ()
    n406 = case shown="True" w629 {
      tunnel: w628 -> [_ w635]
      frame False {
      }
      frame True {
        n407 = call "Z900_navX_Set_ZeroYaw.vi"("navX Device"=w635) -> ()  [unwired: 9 in, 2 out]
      }
    }
  }
  n408 = while {
    tunnel: w20 -> [w679]
    shift-right: [w672] -> _
    shift-left: _ -> [w671]
    shift-left: _ -> [w670]
    shift-left: _ -> [w669]
    shift-left: _ -> [w668]
    shift-left: _ -> [w667]
    shift-left: _ -> [w666]
    shift-left: _ -> [w665]
    shift-left: _ -> [w664]
    shift-left: _ -> [w663]
    shift-left: _ -> [w662]
    shift-left: _ -> [w661]
    shift-left: _ -> [w660]
    shift-left: _ -> [w659]
    shift-left: _ -> [w658]
    shift-left: _ -> [w657]
    shift-left: _ -> [w656]
    shift-left: _ -> [w643]
    shift-left: _ -> [w642]
    shift-left: _ -> [w641]
    shift-left: _ -> [w640]
    shift-left: _ -> [w639]
    stop <- FALSE stop-if-true
    # "Shooter in its own thread to protect everything else"
    # "Yes, I'm reading the encoder\nat 1000 Hz. I don't know how much\nof a difference it makes"
    # "shooter encoder"
    n409 = call <vilib>:"WPI_EncoderGet.vi"("EncoderDevRef"=w679) -> ("Distance"=w677:dbl, "Rate"=w678:dbl)  [unwired: 5 in, 4 out]
    n410 = Build Array(w671, w670, w669, w668, w667, w666, w665, w664, w663, w662, w661, w660, w659, w658, w657, w656, w643, w642, w641, w640, w639) -> (w655:dbl[])
    n411 = Negate(x=w677) -> (-x=w673:dbl)
    n412 = Sort 1D Array(array=w655) -> (sorted array=w654:dbl[])
    n413 = Index Array(array=w654) -> (element #4=w653:dbl, element #5=w652:dbl, element #6=w651:dbl, element #7=w650:dbl, element #8=w649:dbl, element #9=w648:dbl, element #10=w647:dbl, element #11=w646:dbl, element #12=w645:dbl, element #13=w644:dbl, element #14=w638:dbl, element #15=w637:dbl, element #16=w636:dbl)  [unwired: 19 in, 6 out]
    n414 = Compound Arithmetic op=ADD(w653, w652, w651, w650, w649, w648, w647, w646, w645, w644, w638, w637, w636) -> (w676:dbl)
    n415 = Negate(x=w678) -> (-x=w672:dbl)
    n416 = Divide(x=w676, y=13.0) -> (x/y=w674:dbl)
    "Shooter Speed" <- w674
    n417 = global write "Robot Global Data.vi" "encShootPos"(w673) -> ()
    n418 = global write "Robot Global Data.vi" "encShootSpeed"(w674) -> ()
    n419 = Wait (ms)(milliseconds to wait=u32 1) -> ()  [unwired: 1 out]
  }
  n420 = while {
    tunnel: w18 -> [w693]
    tunnel: w16 -> [w692]
    stop <- FALSE stop-if-true
    # "network tables, slow-er sensors"
    n421 = Wait (ms)(milliseconds to wait=u32 20) -> ()  [unwired: 1 out]
    n422 = call <vilib>:"WPI_EncoderGet.vi"("EncoderDevRef"=w693) -> ("Distance"=w690:dbl)  [unwired: 5 in, 5 out]
    n423 = call <vilib>:"WPI_EncoderGet.vi"("EncoderDevRef"=w692) -> ("Distance"=w688:dbl)  [unwired: 5 in, 5 out]
    n424 = Negate(x=w690) -> (-x=w689:dbl)
    n425 = Negate(x=w688) -> (-x=w687:dbl)
    n426 = global write "Robot Global Data.vi" "encXpos"(w689) -> ()
    n427 = global write "Robot Global Data.vi" "encYpos"(w687) -> ()
    n428 = call-poly <vilib>:"NT Read Value.vi"("Name"="target_x") -> ("Numeric"=w685:dbl)  [unwired: 9 in, 1 out]
    n429 = call-poly <vilib>:"NT Read Value.vi"("Name"="battery") -> ("Numeric"=w682:dbl)  [unwired: 9 in, 1 out]
    "voltage dash" <- w682
    n430 = global write "Robot Global Data.vi" "center X"(w685) -> ()
    n431 = global write "Robot Global Data.vi" "Vbat"(w682) -> ()
  }
  n432 = while {
    tunnel: w28 -> [w707]
    stop <- FALSE stop-if-true
    # "hopper"
    n433 = global read "Robot Global Data.vi" "Shot Distance"() -> (w697:bool)
    n434 = global read "Robot Global Data.vi" "Hopper Close"() -> (w699:dbl)
    n435 = Wait (ms)(milliseconds to wait=u32 50) -> ()  [unwired: 1 out]
    n436 = global read "Robot Global Data.vi" "hopper far"() -> (w700:dbl)
    n437 = local read "shooting close"() -> (w695:bool)
    n438 = local read "shooting far"() -> (w696:bool)
    n439 = Select(t=w700, s=w697, f=w699) -> (s? t:f=w701:dbl)
    n440 = global read "Robot Global Data.vi" "Shoot!"() -> (w702:bool)
    n441 = Absolute Value(x=w701) -> (abs(x)=w704:dbl)
    n442 = Or(x=w696, y=w695) -> (x .or. y?=w694:bool)
    n443 = Negate(x=w704) -> (-x=w703:dbl)
    n444 = And(x=w702, y=w694) -> (x .and. y?=w698:bool)
    n445 = Select(t=w703, s=w698, f=0.0) -> (s? t:f=w706:dbl)
    n446 = call <vilib>:"WPI_MotorControlSetOutput.vi"("Output"=w706, "MotorControlDevRef"=w707) -> ()  [unwired: 7 in, 3 out]
  }
  n447 = while {
    stop <- FALSE stop-if-true
    # "I may be overdoing the threads"
    n448 = global read "Robot Global Data.vi" "Trim Far"() -> (w715:dbl)
    n449 = global read "Robot Global Data.vi" "auto"() -> (w718:i32)
    n450 = call-poly <vilib>:"NT Write Value.vi"("Numeric"=w715, "Name"="trim far") -> ()  [unwired: 9 in, 1 out]
    n451 = global read "Robot Global Data.vi" "Trim Close"() -> (w717:dbl)
    n452 = call-poly <vilib>:"NT Write Value.vi"("Numeric"=w718, "Name"="autofeedback") -> ()  [unwired: 9 in, 1 out]
    n453 = call-poly <vilib>:"NT Write Value.vi"("Numeric"=w717, "Name"="trim close") -> ()  [unwired: 9 in, 1 out]
    n454 = call-poly <vilib>:"NT Read Value.vi"("Name"="target_y") -> ("Numeric"=w720:dbl)  [unwired: 9 in, 1 out]
    n455 = global write "Robot Global Data.vi" "center Y"(w720) -> ()
    n456 = call-poly <vilib>:"NT Read Value.vi"("Name"="auto") -> ("Numeric"=w713:dbl)  [unwired: 9 in, 1 out]
    n457 = global write "Robot Global Data.vi" "auto"(w713) -> ()
    n458 = Wait (ms)(milliseconds to wait=u32 100) -> ()  [unwired: 1 out]
  }
  n459 = while {
    stop <- FALSE stop-if-true
    # "These numbers are ones that change frequently enough to be read from the dash.\nMostly autonomous values and shooter values."
    n460 = Wait (ms)(milliseconds to wait=u32 5000) -> ()  [unwired: 1 out]
    n461 = call-poly <vilib>:"NT Read Value.vi"("Name"="fudge values") -> ("Numeric Array"=w764:dbl[])  [unwired: 9 in, 1 out]
    n462 = Index Array(array=w764) -> (element #7=w763:dbl, element #8=w762:dbl, element #9=w761:dbl, element #10=w760:dbl, element #11=w759:dbl, element #12=w758:dbl, element #13=w757:dbl, element #14=w756:dbl, element #15=w755:dbl, element #16=w754:dbl, element #17=w753:dbl, element #18=w752:dbl, element #19=w751:dbl, element #20=w750:dbl, element #21=w749:dbl, element #22=w748:dbl, element #23=w747:dbl, element #24=w746:dbl, element #25=w745:dbl, element #26=w744:dbl, element #27=w743:dbl, element #28=w742:dbl, element #29=w741:dbl, element #30=w738:dbl, element #31=w737:dbl, element #32=w736:dbl, element #33=w735:dbl, element #34=w734:dbl, element #35=w733:dbl, element #36=w732:dbl, element #37=w731:dbl, element #38=w730:dbl, element #39=w729:dbl, element #40=w728:dbl, element #41=w727:dbl, element #42=w726:dbl, element #45=w725:dbl, element #46=w724:dbl, element #47=w723:dbl, element #48=w722:dbl)  [unwired: 48 in, 8 out]
    n463 = global write "Robot Global Data.vi" "auto shot increase power RED"(w726) -> ()
    n464 = global write "Robot Global Data.vi" "auto shot increase time RED"(w727) -> ()
    n465 = global write "Robot Global Data.vi" "auto shot increase power BLUE"(w724) -> ()
    n466 = global write "Robot Global Data.vi" "auto shot increase time BLUE"(w725) -> ()
    n467 = global write "Robot Global Data.vi" "Hopper Far tele"(w763) -> ()
    n468 = global write "Robot Global Data.vi" "Hopper Close"(w762) -> ()
    n469 = global write "Robot Global Data.vi" "Intake Speed"(w761) -> ()
    n470 = global write "Robot Global Data.vi" "Autoaim mid"(w760) -> ()
    n471 = global write "Robot Global Data.vi" "Autoaim fast"(w759) -> ()
    n472 = global write "Robot Global Data.vi" "Autoaim slow"(w758) -> ()
    n473 = global write "Robot Global Data.vi" "FF R60 P2"(w757) -> ()
    n474 = global write "Robot Global Data.vi" "FF R60 P1"(w756) -> ()
    n475 = global write "Robot Global Data.vi" "FF B10 G"(w755) -> ()
    n476 = global write "Robot Global Data.vi" "FF Far Tele"(w754) -> ()
    n477 = global write "Robot Global Data.vi" "FF Close Tele"(w753) -> ()
    n478 = global write "Robot Global Data.vi" "FF B40"(w752) -> ()
    n479 = global write "Robot Global Data.vi" "Camera Target"(w751) -> ()
    n480 = global write "Robot Global Data.vi" "R60P1yDepth"(w750) -> ()
    n481 = global write "Robot Global Data.vi" "R60P2yDepth"(w749) -> ()
    n482 = global write "Robot Global Data.vi" "center gear depth"(w748) -> ()
    n483 = global write "Robot Global Data.vi" "B40yDepth"(w747) -> ()
    n484 = global write "Robot Global Data.vi" "FF R10 G"(w746) -> ()
    n485 = global write "Robot Global Data.vi" "gearDepthThresh"(w745) -> ()
    n486 = global write "Robot Global Data.vi" "gearSensThresh"(w744) -> ()
    n487 = global write "Robot Global Data.vi" "PID close shot target"(w743) -> ()
    n488 = global write "Robot Global Data.vi" "PID far shot target"(w742) -> ()
    n489 = global write "Robot Global Data.vi" "Shooter \"i\""(w741) -> ()
    n490 = global write "Robot Global Data.vi" "R60P2 shotEnc"(w738) -> ()
    n491 = global write "Robot Global Data.vi" "R60P1 shotEnc"(w737) -> ()
    n492 = global write "Robot Global Data.vi" "B40P1 shotEnc"(w736) -> ()
    n493 = global write "Robot Global Data.vi" "B10G shotEnc"(w735) -> ()
    n494 = global write "Robot Global Data.vi" "R10G shotEnc"(w734) -> ()
    n495 = global write "Robot Global Data.vi" "R60P2 X"(w733) -> ()
    n496 = global write "Robot Global Data.vi" "R60P1 X"(w732) -> ()
    n497 = global write "Robot Global Data.vi" "B40 X"(w731) -> ()
    n498 = global write "Robot Global Data.vi" "R60P2 y pullup"(w730) -> ()
    n499 = global write "Robot Global Data.vi" "R60P1 y pullup"(w729) -> ()
    n500 = global write "Robot Global Data.vi" "B40 y pullup"(w728) -> ()
    n501 = global write "Robot Global Data.vi" "no trigger pullback"(w722) -> ()
    n502 = global write "Robot Global Data.vi" "no trigger y depth"(w723) -> ()
  }
